vi "UT_Main.vi"(8 "error in":errorcluster, 10 "Report Path":path, 11 "Interactive":bool) -> (0 "error out":errorcluster)   [LabVIEW 2020]
doc: "Main VI for all unit tests. All unit test VIs are hierachically called from this VI."
uses:
  <vilib>/addons/_JKI Toolkits/Caraya/classes/Test Suite/Define Test Suite (SimpleText Report).vi
  <vilib>/addons/_JKI Toolkits/Caraya/classes/Test Suite/Test Suite.lvclass
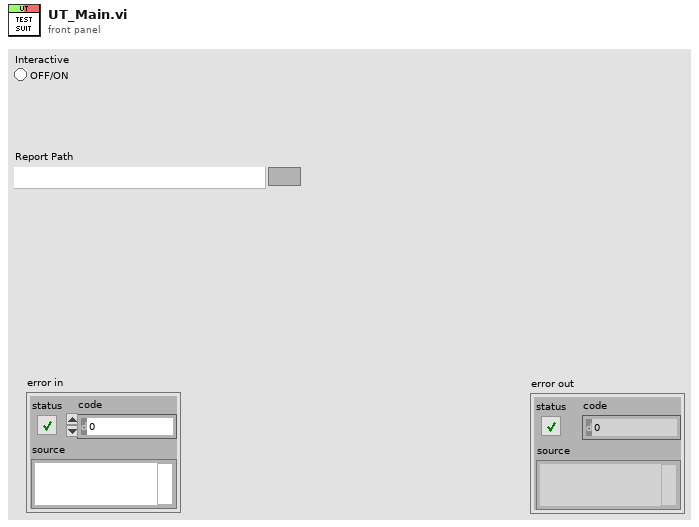
[diagram p1: front panel]
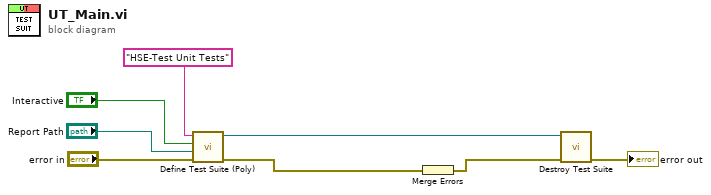
[diagram p0: block diagram]
diagram:
  n1 = call-poly <vilib>:"Define Test Suite (Poly).vi"("error in (no error)"="error in", "Report Path"="Report Path", "Interactive"="Interactive", "Label (VI Title)"="HSE-Test Unit Tests") -> ("error out"=w1:errorcluster, "Test Suite"=w3:refnum<class "Test Suite.lvclass">)  [unwired: 5 in, 1 out]
  n2 = Merge Errors(w1) -> (w4:errorcluster)
  n3 = call-dynamic "Destroy Test Suite.vi"("error in (no error)"=w4, "Test Suite in"=w3) -> ("error out"=→"error out":errorcluster)  [unwired: 8 in, 1 out]
